vi "Agilent 34401 Read Transient Measurement.vi"() -> ()   [LabVIEW 2013]
doc: "This example shows how to configure a measurement and take a transient reading.\n\n<B>Note:</B>\n\n(1) This VI only applies to the Agilent 34410/34411 models.\n\n(2) This VI only supports DC/AC current and voltage measurements."
uses:
  <vilib>/Utility/error.llb/DialogType.ctl
  <instrlib>/Agilent 34401/Public/Data/Read (Transient).vi
  <instrlib>/Agilent 34401/Agilent 34401.lvlib
panel:
  out "Peak-to-Peak":dbl
  out "Minimum":dbl
  out "Maximum":dbl
  in  "Function (0: DC Voltage)":u16(ring) items=["DC Voltage", "AC Voltage", "2 - Wire Resistance", "4 - Wire Resistance", "DC Current", "AC Current", "Frequency", "Period", "Continuity", "Diode Checking", "VDC:VDC Ratio", "Temperature", "Capacitance"]
  in  "Enable Auto Range (T: Enable)":bool=TRUE
  in  "Manual Resolution (5.5 Digits)":dbl(ring)=5.5 items=["4.5"=4.5, "5.5"=5.5, "6.5"=6.5]
  in  "Manual Range (1.00)":dbl=1.0 format="%_3f"
  out "Measurement":dbl
  in  "VISA resource name":refnum<visa-resource-name>
  # "(c) 2005-2008 National Instruments.  ALL RIGHTS RESERVED."
  # "Note: This VI only applies to the Agilent 34410/34411 models.\nOnly AC/DC current and voltage measurements apply"
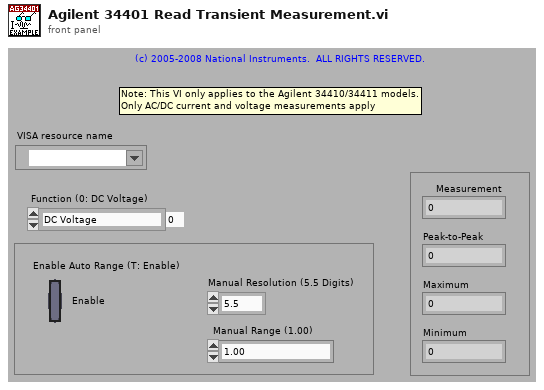
[diagram p1: front panel]
types:
  T1 = typedef "DialogType.ctl" = u16
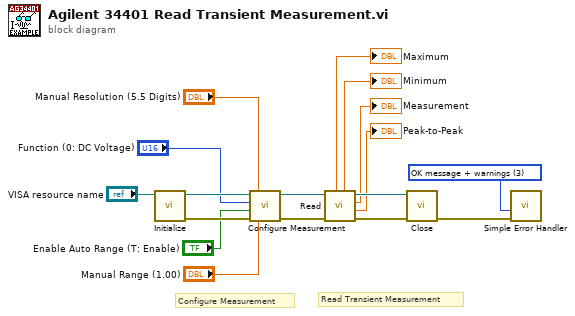
[diagram p0: block diagram]
diagram:
  w2 = T1 3 items=["no dialog", "OK message", "continue or stop message", "OK message + warnings", "continue/stop + warnings"] ("type of dialog (OK msg:1)")
  # "Read Transient Measurement"
  # "Configure Measurement"
  n1 = call <instrlib>:"Initialize.vi"("VISA resource name"="VISA resource name") -> ("error out"=w9:errorcluster, "VISA resource name out"=w10:refnum<visa-resource-name>)  [unwired: 9 in]
  n2 = call <instrlib>:"Configure Measurement.vi"("Manual Range (1.00)"="Manual Range (1.00)", "Manual Resolution (5.5 Digits)"="Manual Resolution (5.5 Digits)", "error in (no error)"=w9, "Enable Auto Range (T: Enable)"="Enable Auto Range (T: Enable)", "Function (0: DC Voltage)"="Function (0: DC Voltage)", "VISA resource name"=w10) -> ("error out"=w11:errorcluster, "VISA resource name out"=w12:refnum<visa-resource-name>)  [unwired: 4 in]
  n3 = call-poly <instrlib>:"Read.vi"("error in (no error)"=w11, "VISA resource name"=w12) -> ("error out"=w15:errorcluster, "Peak-to-Peak"=→"Peak-to-Peak":dbl, "Measurement"=→"Measurement":dbl, "VISA resource name out"=w14:refnum<visa-resource-name>, "Minimum"=→"Minimum":dbl, "Maximum"=→"Maximum":dbl)  [unwired: 4 in]
  n4 = call <instrlib>:"Close.vi"("error in (no error)"=w15, "VISA resource name"=w14) -> ("error out"=w17:errorcluster)  [unwired: 9 in]
  n5 = call <vilib>:"Simple Error Handler.vi"("type of dialog (OK msg:1)"=w2, "error in (no error)"=w17) -> ()  [unwired: 3 in, 5 out]
